vi "PNS Testversuch.vi"() -> ()   [LabVIEW 2020, in "PNS.lvlib"]
uses:
  PNS.lvlib
panel:
  in  "String":string
  out "Nach Teil-String":string
  out "Vor Teil-String":string
  in  "Eingang":dbl
  out "Ausgang":dbl
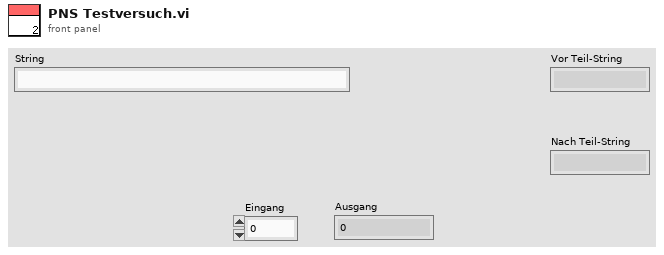
[diagram p1: front panel]
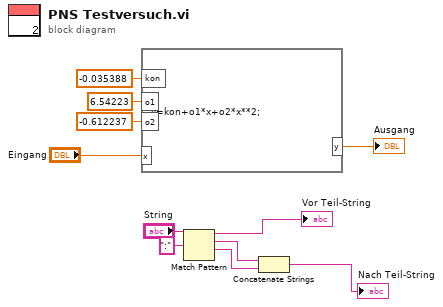
[diagram p0: block diagram]
diagram:
  n1 = formula code="y=kon+o1*x+o2*x**2;"("x"="Eingang", "kon"=-0.035388 ("Eingangsvariable"), "o1"=6.54223 ("Eingangsvariable"), "o2"=-0.612237 ("Eingangsvariable")) -> ("y"=→"Ausgang":dbl)
  n2 = Match Pattern(string="String", regular expression=":" ("Regulärer Ausdruck")) -> (before substring=→"Vor Teil-String":string, match substring=w3:string, after substring=w2:string)  [unwired: 1 in, 1 out]
  n3 = Concatenate Strings(w3, w2) -> (→"Nach Teil-String":string)
